vi "convertVecToArray_bin_01.vi"(1 "data":i16[](array[numeric]), 2 "Channels to read":i32=6) -> (0 "transposed array":dbl[][](array[numeric]))   [LabVIEW 2021]
uses:
  <userlib>/er4_163/er4commlib_labview.lvlib
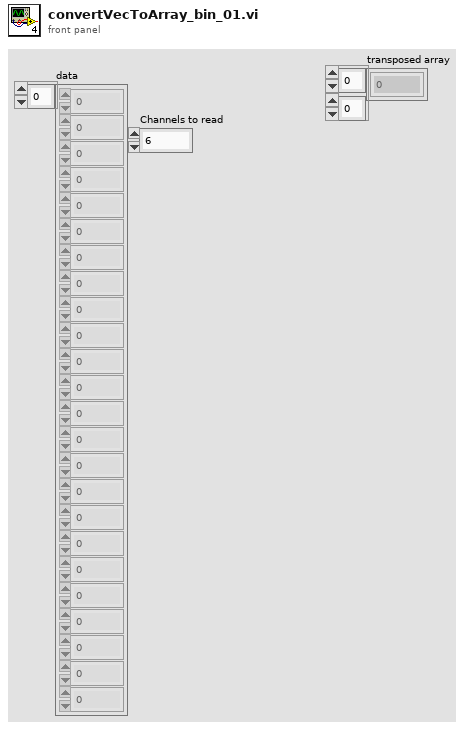
[diagram p1: front panel]
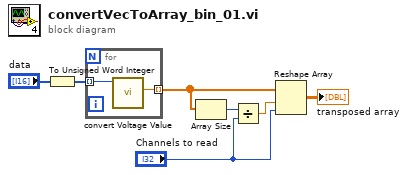
[diagram p0: block diagram]
diagram:
  n1 = To Unsigned Word Integer(number="data") -> (unsigned 16bit integer=w3:u16[])
  n2 = for {
    tunnel: w3 -> [w9] mode=indexing
    tunnel: [w8] -> w7 mode=indexing
    n3 = call <userlib>:"convert Voltage Value.vi"("intValue"=w9) -> ("fltValue out"=w8:dbl)  [unwired: 8 in, 2 out]
  }
  n4 = Array Size(array=w7) -> (size(s)=w4:i32)
  n5 = Divide(x=w4, y="Channels to read") -> (x/y=w5:dbl)
  n6 = Reshape Array(w7, w5, "Channels to read") -> (→"transposed array":dbl[][])
